vi "StrConcat.vi"(8 "error in":errorcluster caption="错误输入", 11 "StrArray":string[](array[string])) -> (0 "error out":errorcluster caption="错误输出", 3 "StrOut":string)   [LabVIEW 2013]
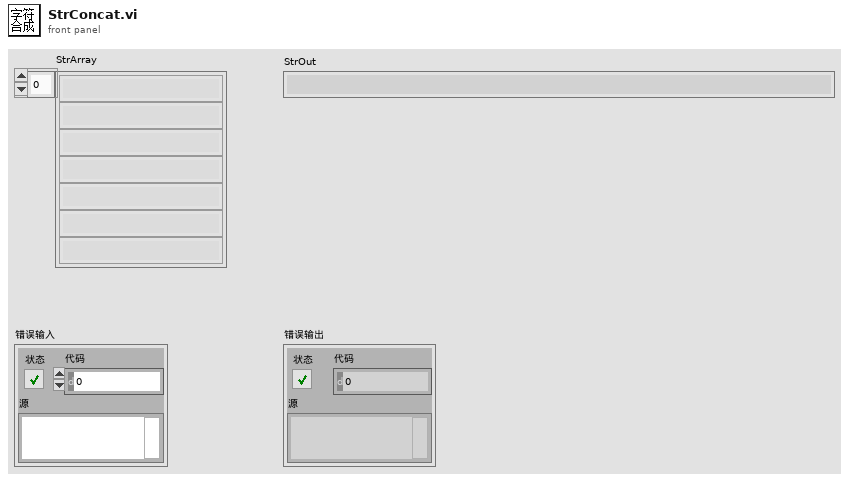
[diagram p1: front panel]
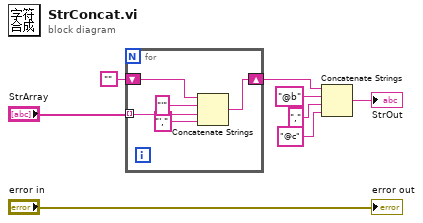
[diagram p0: block diagram]
diagram:
  n1 = for {
    shift-right: [w13] -> w6
    shift-left: "" -> [w12]
    tunnel: "StrArray" -> [w9] mode=indexing
    n2 = Concatenate Strings(w12, "'", w9, "',") -> (w13:string)
  }
  n3 = Concatenate Strings(w6, "@b", ",", "@c") -> (→"StrOut":string)
  "error out" <- "error in"
